vi "State_Machine.vi"(8 "error in (no error)":errorcluster caption="entrée d'erreur (pas d'erreur)", 11 "Get_Voltage en entrée":refnum<class "Get_Addr_Mac_DB_AIS.lvclass">) -> (0 "error out":errorcluster caption="sortie d'erreur", 2 "Json_String":string, 3 "Get_Voltage en sortie":refnum<class "Get_Addr_Mac_DB_AIS.lvclass">)   [LabVIEW 2020, in "Library Test.lvlib" / "Get_Addr_Mac_DB_AIS.lvclass"]
uses:
  Get_Addr_Mac_DB_AIS.lvclass
  C:/Users/ngarcin/OneDrive - Altyor/Standard TB/Suite TB45/Class/Test/Find_SN_In_Database/Find_SN_In_Database.lvclass
  C:/Users/ngarcin/OneDrive - Altyor/Standard TB/Suite TB45/Class/Test/Test (Default)/Test (Default).lvclass
  Commun VI/TypeDef/Variable Printable.ctl
  JSON API/JSON Value/Set from JSON string.vi
  JSON API/JSON Value/JSON Value.lvclass
  Find_SN_In_Database/Find_SN_In_Database.lvclass
  Commun VI/Library Commun.lvlib
  JSON API/Variant JSON/Variant JSON.lvlib
  JSON API/Get Polymorphic/JSON GetSet.lvlib
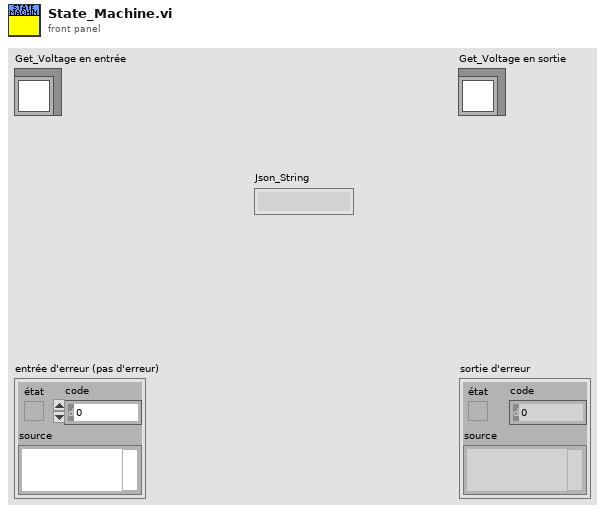
[diagram p1: front panel]
types:
  T1 = typedef "Variable Printable.ctl" = string
  T2 = enum16{"Get Variable", "Get All Variables", "Set Variable", "Delete Variable", "Delete All Variable"}
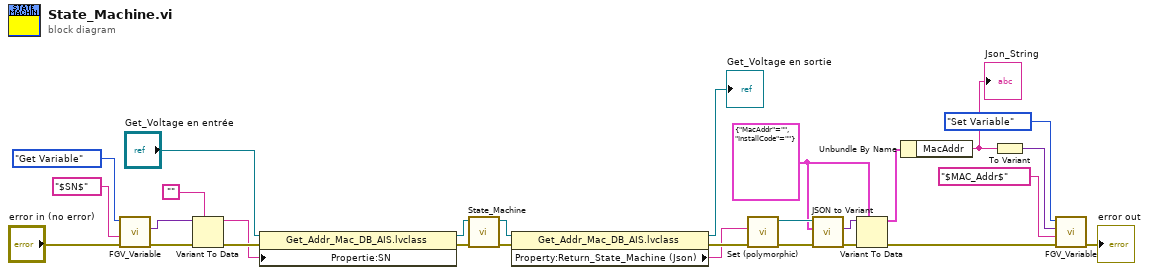
[diagram p0: block diagram]
diagram:
  w17 = cluster{"MacAddr":string, "InstallCode":string} {"MacAddr"="", "InstallCode"=""}
  n1 = call "FGV_Variable.vi"("error in (no error)"="error in (no error)", "Variable"=T1 "$SN$", "Function"=T2."Get Variable") -> ("error out"=w10:errorcluster, "Data Out"=w9:variant)  [unwired: 6 in, 1 out]
  n2 = Variant To Data(error in=w10, type="", Variant=w9) -> (data=w1:string, error out=w7:errorcluster)
  n3 = property class="Get_Addr_Mac_DB_AIS.lvclass"(reference="Get_Voltage en entrée", error in=w7, "Propertie:SN"=w1) -> (reference out=w5:refnum<class "Get_Addr_Mac_DB_AIS.lvclass">, error out=w3:errorcluster)
  n4 = call-parent "State_Machine.vi"("error in (no error)"=w3, "Generate_SN en entrée"=w5) -> ("error out"=w23:errorcluster, "Generate_SN en sortie"=w22:refnum<class "Get_Addr_Mac_DB_AIS.lvclass">)  [unwired: 7 in, 1 out]
  n5 = property class="Get_Addr_Mac_DB_AIS.lvclass"(reference=w22, error in=w23) -> (reference out=→"Get_Voltage en sortie":refnum<class "Get_Addr_Mac_DB_AIS.lvclass">, error out=w15:errorcluster, "Property:Return_State_Machine (Json)"=w12:string)
  n6 = call-poly "Set (polymorphic).vi"("error in (no error)"=w15, "JSON stream"=w12) -> ("error out"=w20:errorcluster, "JSON Value out"=w18:refnum<class "JSON Value.lvclass">)  [unwired: 7 in, 1 out]
  n7 = call "JSON to Variant.vi"("error in (no error)"=w20, "Variant (Data Type)"=w17, "JSON Value"=w18) -> ("error out"=w19:errorcluster, "Variant out"=w21:variant)  [unwired: 7 in]
  n8 = Variant To Data(error in=w19, type=w17, Variant=w21) -> (data=w16:cluster{"MacAddr":string, "InstallCode":string}, error out=w14:errorcluster)
  n9 = Unbundle By Name(w16) -> ("MacAddr"=w13:string)
  "Json_String" <- w13
  n10 = To Variant(anything=w13) -> (Variant=w27:variant)
  n11 = call "FGV_Variable.vi"("error in (no error)"=w14, "Variable"=T1 "$MAC_Addr$" ("Variable Printable"), "Data In"=w27, "Function"=T2."Set Variable") -> ("error out"=→"error out":errorcluster)  [unwired: 5 in, 2 out]
